vi "Self Catch.vi"(6 "reinit?":bool) -> (0 "Low Gear":bool, 1 "Y":dbl, 3 "X steer":dbl)   [LabVIEW 2013]
uses:
  Common Code/Change Detect Boolean.vi
  Robot Global Data.vi
  <vilib>/Rock Robotics/WPI/Gyro/WPI_GyroRefNum Registry Get.vi
  <vilib>/Rock Robotics/WPI/Gyro/WPI_GyroGetAngle.vi
panel:
  out "X":dbl
  in  "Heading":dbl
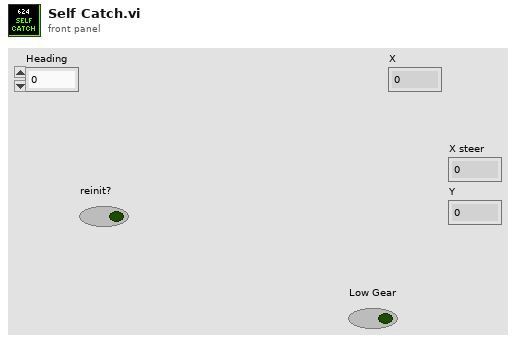
[diagram p1: front panel]
types:
  T1 = cluster{"X Dist":cluster{"PID gains":cluster{"proportional gain (Kc)":dbl, "integral time (Ti, min)":dbl, "derivative time (Td, min)":dbl}, "output range":cluster{"output high":dbl, "output low":dbl}}, "Y Dist":cluster{"PID gains":cluster{"proportional gain (Kc)":dbl, "integral time (Ti, min)":dbl, "derivative time (Td, min)":dbl}, "output range":cluster{"output high":dbl, "output low":dbl}}}
  T2 = cluster{"proportional gain (Kc)":dbl, "integral time (Ti, min)":dbl, "derivative time (Td, min)":dbl}
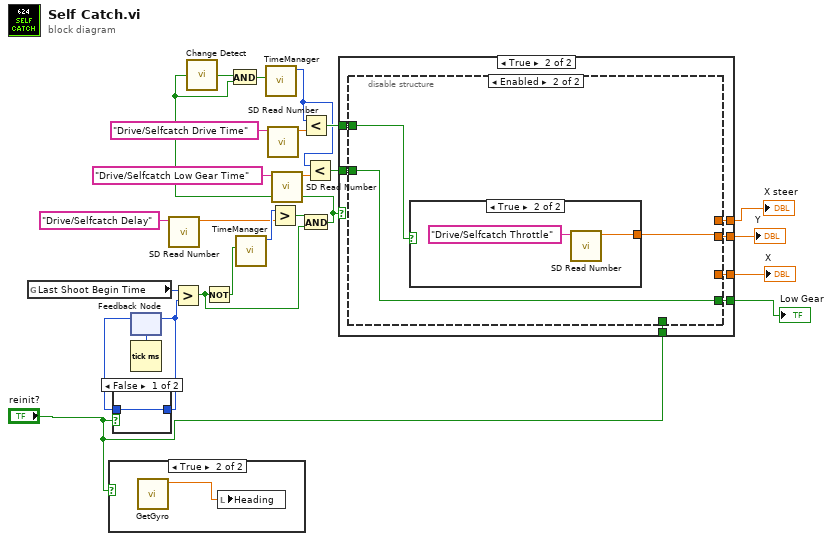
[diagram p0: block diagram]
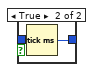
[diagram p3: hidden frame]
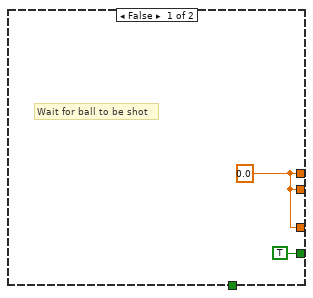
[diagram p4: hidden frame]
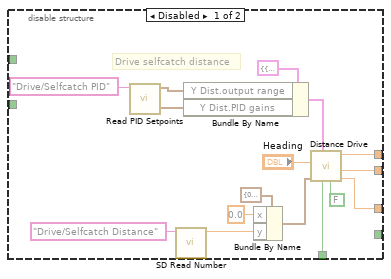
[diagram p5: hidden frame]
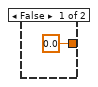
[diagram p6: hidden frame]
diagram:
  n1 = global read "Robot Global Data.vi" "Last Shoot Begin Time"() -> (w19:u32)
  n2 = case shown="True" "reinit?" {
    frame False {
    }
    frame True {
      n3 = call "GetGyro.vi"() -> ("Angle"=w26:dbl)  [unwired: 9 in, 2 out]
      n4 = local write "Heading"(w26) -> ()
    }
  }
  n5 = Tick Count (ms)() -> (millisecond timer value=w23:u32)
  n6 = feedback #1(w23) -> (w22:u32)
  n7 = case shown="False" "reinit?" {
    tunnel: w22 -> [w27 _]
    tunnel: [w27 w28] -> w21
    frame False {
    }
    frame True {
      n8 = Tick Count (ms)() -> (millisecond timer value=w28:u32)
    }
  }
  n9 = feedback-in #1(w21) -> ()
  n10 = call <vilib>:"SD Read Number.vi"("Name"="Drive/Selfcatch Delay") -> ("Numeric"=w15:dbl)  [unwired: 8 in, 2 out]
  n11 = Greater?(x=w19, y=w21) -> (0:w13:bool)
  n12 = Not(x=w13) -> (.not. x?=w17:bool)
  n13 = call "TimeManager.vi"("Reset?"=w17) -> ("Time Since Reset"=w16:u32)  [unwired: 9 in, 1 out]
  n14 = call <vilib>:"SD Read Number.vi"("Name"="Drive/Selfcatch Drive Time") -> ("Numeric"=w7:dbl)  [unwired: 8 in, 2 out]
  n15 = Greater?(x=w16, y=w15) -> (0:w14:bool)
  n16 = call <vilib>:"SD Read Number.vi"("Name"="Drive/Selfcatch Low Gear Time") -> ("Numeric"=w4:dbl)  [unwired: 8 in, 2 out]
  n17 = And(x=w14, y=w13) -> (x .and. y?=w9:bool)
  n18 = call-poly "Change Detect.vi"("In"=w9) -> ("Changed?"=w10:bool)
  n19 = And(x=w10, y=w9) -> (x .and. y?=w8:bool)
  n20 = call "TimeManager.vi"("Reset?"=w8) -> ("Time Since Reset"=w3:u32)  [unwired: 9 in, 1 out]
  n21 = Less?(x=w3, y=w7) -> (x < y?=w5:bool)
  n22 = Less?(x=w3, y=w4) -> (x < y?=w1:bool)
  n23 = case shown="True" w9 {
    tunnel: [w30 w37] -> w25
    tunnel: [w30 w36] -> w24
    tunnel: "reinit?" -> [_ w35]
    tunnel: [w30 w34] -> w12
    tunnel: w5 -> [_ w33]
    tunnel: [TRUE w32] -> w2
    tunnel: w1 -> [_ w31]
    frame False {
      w30 = 0.0 ("X steer")
      # "Wait for ball to be shot"
    }
    frame True {
      n24 = disable-structure shown="Enabled" {
        disable-tunnel: [w50 _] -> w37
        disable-tunnel: [w49 w56] -> w36
        disable-tunnel: w35 -> [w48 _]
        disable-tunnel: [w38 _] -> w34
        disable-tunnel: w33 -> [_ w55]
        disable-tunnel: [_ w54] -> w32
        disable-tunnel: w31 -> [_ w54]
        frame Disabled {
          # "Drive selfcatch distance"
          n25 = call "Read PID Setpoints.vi"("SD Name"="Drive/Selfcatch PID" ("Name")) -> ("PID gains"=w53:T2, "output range"=w45:cluster{"output high":dbl, "output low":dbl})  [unwired: 9 in]
          n26 = call <vilib>:"SD Read Number.vi"("Name"="Drive/Selfcatch Distance") -> ("Numeric"=w41:dbl)  [unwired: 8 in, 2 out]
          n27 = Bundle By Name(cluster=T1 {"X Dist"={"PID gains"={"proportional gain (Kc)"=0.0, "integral time (Ti, min)"=0.0, "derivative time (Td, min)"=0.0}, "output range"={"output high"=0.0, "output low"=0.0}}, "Y Dist"={"PID gains"={"proportional gain (Kc)"=0.0, "integral time (Ti, min)"=0.0, "derivative time (Td, min)"=0.0}, "output range"={"output high"=0.0, "output low"=0.0}}} ("PID Params"), "Y Dist.output range"=w45, "Y Dist.PID gains"=w53) -> (w44:T1)
          n28 = Bundle By Name(cluster=cluster{"x":dbl, "y":dbl} {"x"=0.0, "y"=0.0} ("distance target"), "x"=0.0, "y"=w41) -> (w42:cluster{"x":dbl, "y":dbl})
          n29 = call "Distance Drive.vi"("omni?"=FALSE, "reinit?"=w48, "PID Params"=w44, "distance target"=w42, "Heading"="Heading") -> ("X"=w38:dbl, "Y"=w49:dbl, "X steer"=w50:dbl)  [unwired: 4 in]
        }
        frame Enabled {
          n30 = case shown="True" w55 {
            tunnel: [0.0 ("Numeric") w58] -> w56
            frame False {
            }
            frame True {
              n31 = call <vilib>:"SD Read Number.vi"("Name"="Drive/Selfcatch Throttle") -> ("Numeric"=w58:dbl)  [unwired: 8 in, 2 out]
            }
          }
        }
      }
    }
  }
  "X steer" <- w25
  "Y" <- w24
  "X" <- w12
  "Low Gear" <- w2
